vi "Get Data Name From TD.vi"(8 "错误输入":errorcluster, 10 "Type Descriptor":u16[](array[numeric]) format="%.0x") -> (0 "错误输出":errorcluster, 2 "Name":string)   [LabVIEW 2012, in "TD Tools.lvlib"]
uses:
  TD Tools.lvlib
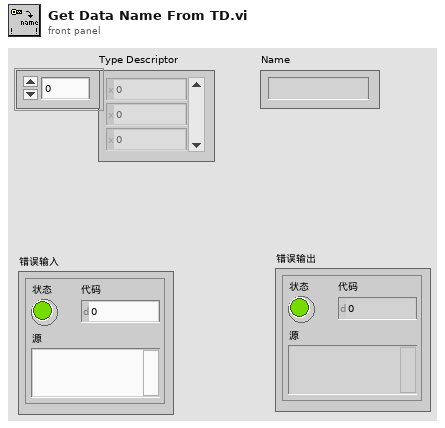
[diagram p1: front panel]
types:
  T1 = typedef "TD Tools.lvlib/Type Descriptor Header.ctl" = cluster{"length":u16, "private":u8, "type":T2, "# elements":u16}
  T2 = typedef "TD Tools.lvlib/Type Descriptor Enumeration.ctl" = enum16{"<Null>", "I8", "I16", "I32", "I64", "U8", "U16", "U32", "U64", "SGL", "DBL", "EXT", "CSG", "CDB", "CXT", "0x0F", "0x10", "0x11", "0x12", "0x13", "0x14", "Enum U8", "Enum U16", "Enum U32", "Enum U64", "SGL PQ", "DBL PQ", "EXT PQ", "CSG PQ", "CDB PQ", "CXT PQ", "0x1F", "0x20", "Boolean", "0x22", "0x23", "0x24", "0x25", "0x26", "0x27", "0x28", "0x29", "0x2A", "0x2B", "0x2C", "0x2D", "0x2E", "0x2F", "String", "0x31", "Path", "Pict", "0x34", "0x35", "0x36", "DAQ", "0x38", "0x39", "0x3A", "0x3B", "0x3C", "0x3D", "0x3E", "0x3F", "Array", "0x41", "0x42", "0x43", "0x44", "0x45", "0x46", "0x47", "0x48", "0x49", "0x4A", "0x4B", "0x4C", "0x4D", "0x4E", "0x4F", "Cluster", "0x51", "0x52", "Variant", "Waveform", "0x55", "0x56", "0x57", "0x58", "0x59", "0x5A", "0x5B", "0x5C", "0x5D", "0x5E", "0x5F", "0x60", "0x61", "0x62", "0x63", "0x64", "0x65", "0x66", "0x67", "0x68", "0x69", "0x6A", "0x6B", "0x6C", "0x6D", "0x6E", "0x6F", "Refnum"}
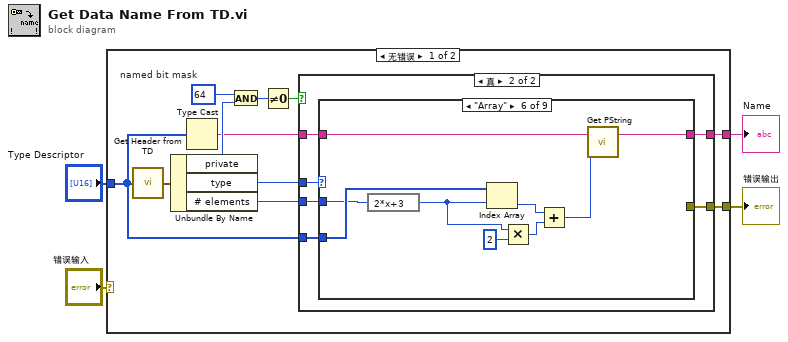
[diagram p0: block diagram]
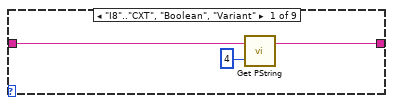
[diagram p3: hidden frame]
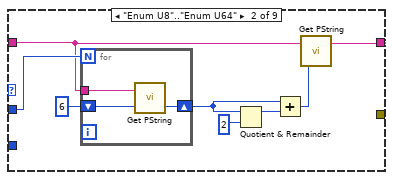
[diagram p4: hidden frame]
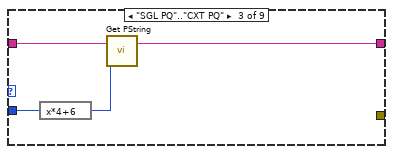
[diagram p5: hidden frame]
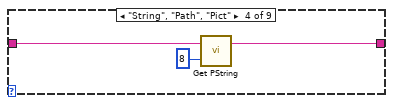
[diagram p6: hidden frame]
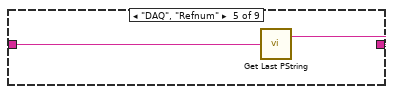
[diagram p7: hidden frame]
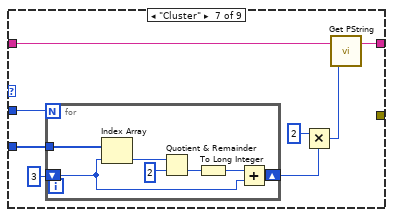
[diagram p8: hidden frame]
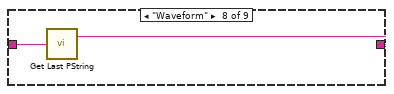
[diagram p9: hidden frame]
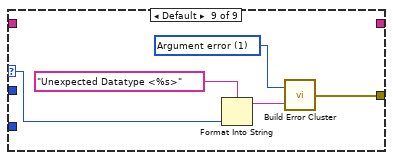
[diagram p10: hidden frame]
diagram:
  n1 = case shown="无错误" "错误输入" {
    selector: "错误输入" -> [_ w76]
    tunnel: "Type Descriptor" -> [w8 _]
    tunnel: [w10 _] -> w2
    tunnel: [w5 w76] -> w1
    frame No Error {
      w14 = u8 64  # named bit mask
      n2 = call "Get Header from TD.vi"("Type Desciptor"=w8) -> ("Type Descriptor Header"=w15:T1)
      n3 = Unbundle By Name(w15) -> ("private"=w13:u8, "type"=w9:T2, "# elements"=w6:u16)
      n4 = Type Cast(x=w8) -> (*(type *) &x=w7:string)  [unwired: 1 in]
      n5 = And(x=w14, y=w13) -> (x .and. y?=w12:u8)
      n6 = Not Equal To 0?(x=w12) -> (x != 0?=w11:bool)
      n7 = case shown="真" w11 {
        tunnel: [_ w19] -> w10
        tunnel: w9 -> [_ w21]
        tunnel: w8 -> [_ w20]
        tunnel: w7 -> [_ w17]
        tunnel: w6 -> [_ w18]
        tunnel: [_ w16] -> w5
        frame False {
        }
        frame True {
          n8 = case shown="\"Array\"" w21 {
            selector: w21 -> [_ _ _ _ _ _ _ _ w74]
            tunnel: w20 -> [_ _ _ _ _ w52 w61 _ _]
            tunnel: w17 -> [w24 w26 w37 w42 w44 w53 w55 w70 _]
            tunnel: [w22 w25 w36 w41 w43 w46 w54 w69 _] -> w19
            tunnel: w18 -> [_ w32 w39 _ _ w51 w59 _ _]
            tunnel: [_ _ _ _ _ _ _ _ w71] -> w16
            frame "I8".."CXT", "Boolean", "Variant" {
              n9 = call "Get PString.vi"("offset(0)"=4, "String"=w24) -> ("PString"=w22:string)  [unwired: 1 out]
            }
            frame "Enum U8".."Enum U64" {
              n10 = for {
                N: w32 -> [_]
                shift-right: [w33] -> w28
                shift-left: 6 ("offset  Past PString") -> [w34]
                tunnel: w26 -> [w35]
                n11 = call "Get PString.vi"("offset(0)"=w34, "String"=w35) -> ("offset  Past PString"=w33:i32)  [unwired: 1 out]
              }
              n12 = Quotient & Remainder(x=w28, y=2) -> (x-y*floor(x/y)=w30:i32)  [unwired: 1 out]
              n13 = Add(x=w28, y=w30) -> (x+y=w27:i32)
              n14 = call "Get PString.vi"("offset(0)"=w27, "String"=w26) -> ("PString"=w25:string)  [unwired: 1 out]
            }
            frame "SGL PQ".."CXT PQ" {
              n15 = expression code="x*4+6"(w39) -> (w38:u16)
              n16 = call "Get PString.vi"("offset(0)"=w38, "String"=w37) -> ("PString"=w36:string)  [unwired: 1 out]
            }
            frame "String", "Path", "Pict" {
              n17 = call "Get PString.vi"("offset(0)"=8, "String"=w42) -> ("PString"=w41:string)  [unwired: 1 out]
            }
            frame "DAQ", "Refnum" {
              n18 = call "Get Last PString.vi"("String"=w44) -> ("Last String"=w43:string)  [unwired: 1 out]
            }
            frame "Array" {
              n19 = expression code="2*x+3"(w51) -> (w45:u16)
              n20 = Index Array(array=w52, index=w45) -> (element=w48:u16)
              n21 = Multiply(x=w45, y=u16 2) -> (x*y=w49:u16)
              n22 = Add(x=w48, y=w49) -> (x+y=w47:u16)
              n23 = call "Get PString.vi"("offset(0)"=w47, "String"=w53) -> ("PString"=w46:string)  [unwired: 1 out]
            }
            frame "Cluster" {
              n24 = for {
                N: w59 -> [_]
                shift-right: [w67] -> w58
                shift-left: 3 -> [w66]
                tunnel: w61 -> [w68]
                n25 = Index Array(array=w68, index=w66) -> (element=w64:u16)
                n26 = Quotient & Remainder(x=w64, y=i16 2) -> (floor(x/y)=w65:u16)  [unwired: 1 out]
                n27 = To Long Integer(number=w65) -> (32bit integer=w62:i32)
                n28 = Add(x=w62, y=w66) -> (x+y=w67:i32)
              }
              n29 = Multiply(x=2 ("y"), y=w58) -> (x*y=w56:i32)
              n30 = call "Get PString.vi"("offset(0)"=w56, "String"=w55) -> ("PString"=w54:string)  [unwired: 1 out]
            }
            frame "Waveform" {
              n31 = call "Get Last PString.vi"("String"=w70) -> ("Last String"=w69:string)  [unwired: 1 out]
            }
            frame Default {
              w73 = 1 items=["No error", "Argument error", "Memory is full", "Out of zone", "End of file", "File already open", "Generic file I/O error", "File not found", "File permission error", "Disk is full", "Duplicate path", "Too many files open", "System feature not enabled", "Resource file not found", "Cannot add resource", "Resource not found", "Image not found", "Image memory error", "Pen does not exist", "Config type invalid", "Config token not found", "Config parse error", "Config memory error", "Bad external code format", "Bad external code offset", "External code not present", "Null window", "Destroy window error", "Null menu", "Print aborted", "Bad print record", "Print driver error", "Windows error during printing", "Memory error during printing", "Print dialog error", "Generic print error", "Invalid device refnum", "Device not found", "Device parameter error", "Device unit error", "Cannot open device", "Device call aborted", "Generic error", "Cancelled by user", "Object ID too low", "Object ID too high", "Object not in heap", "Unknown heap", "Unknown object (invalid DefProc)", "Unknown object (DefProc not in table)", "Message out of range", "Invalid (null) method", "Unknown message", "Manager call not supported", "Bad address", "Network operation in progress", "Network operation timed out", "Connection is busy", "Network attribute not supported", "Network error", "Address in use", "System out of memory", "Connection aborted", "Connection refused", "Not connected", "Already connected", "Connection closed", "Initialization error (interapplication manager)", "Bad occurrence", "Wait on unbound occurrence handler", "Occurrence queue overflow", "Datalog type conflict", "Unused", "Unrecognized type (interapplication manager)", "Memory corrupt", "Failed to make temporary DLL", "Old CIN version", "Drag socket not found", "Failed to load drop-object", "Failed to register OLE object", "Failed to release OLE object", "Format specifier type mismatch", "Unknown format specifier", "Too few format specifiers", "Too many format specifiers", "Scan failed", "Newer CIN version", "Error converting to variant", "Runtime menu error", "Password tampered", "Variant attribute not found", "Incompatible variant data type", "Event data is not available", "Event Store is not present", "Occurrence is not found", "Event Queue is not created", "Event info is not available", "Refnum passed is NULL", "Error retrieving Class GUID", "Error retrieving CoClass GUID", "Error retrieving TypeLib GUID.", "Bad built application magic bytes.", "Specific driver is different from the specific driver associated with the Logical Name.", "There is no session opened to the class driver.", "Max Error", "MAX - Error with config objects", "MAX - Error loading configuration", "MAX - Group not supported"]
              n32 = Format Into String(format string="Unexpected Datatype <%s>" ("Format String"), w74) -> (resulting string=w72:string)  [unwired: 2 in, 1 out]
              n33 = call "Build Error Cluster.vi"("String to Prepend to source (\"\")"=w72, "code"=w73) -> ("error out"=w71:errorcluster)
            }
          }
        }
      }
    }
    frame Error {
    }
  }
  "Name" <- w2
  "错误输出" <- w1
